vi "dane_do_wykresu.vi"() -> ()   [LabVIEW 2018]
uses:
  <vilib>/Utility/file.llb/Read Delimited Spreadsheet (string).vi
panel:
  out "Mixed Signal Graph":dbl[][](graph)
  in  "Path":path
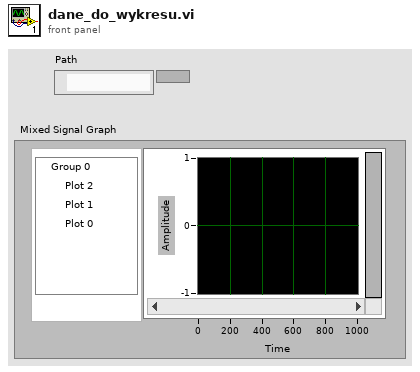
[diagram p1: front panel]
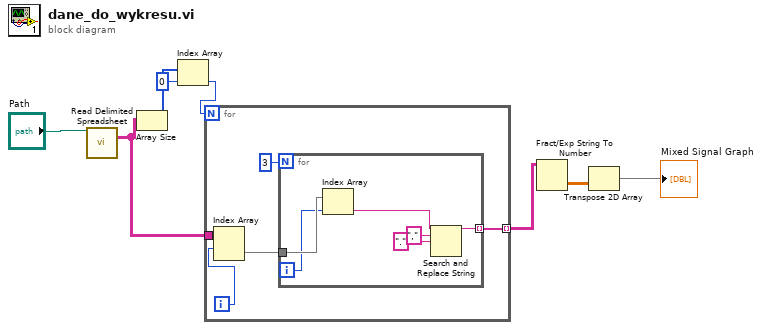
[diagram p0: block diagram]
diagram:
  n1 = call-poly <vilib>:"Read Delimited Spreadsheet.vi"("file path (dialog if empty)"="Path") -> ("all rows"=w2:string[][])  [unwired: 9 in, 5 out]
  n2 = Array Size(array=w2) -> (size(s)=w6:i32[])
  n3 = Index Array(array=w6, index=0) -> (element=w5:i32)
  n4 = for {
    N: w5 -> [_]
    tunnel: [w13] -> w3 mode=indexing
    tunnel: w2 -> [w11]
    i -> [w10]
    n5 = Index Array(array=w11, index (row)=w10) -> (element=w9:string[])  [unwired: 1 in]
    n6 = for {
      N: 3 -> [_]
      tunnel: [w17] -> w13 mode=indexing
      tunnel: w9 -> [w16]
      i -> [w15]
      n7 = Index Array(array=w16, index=w15) -> (element=w14:string)
      n8 = Search and Replace String(input string=w14, search string=",", replace string="." ("replace string (\"\")")) -> (result string=w17:string)  [unwired: 5 in, 3 out]
    }
  }
  n9 = Fract/Exp String To Number(string=w3) -> (number=w7:dbl[][])  [unwired: 3 in, 1 out]
  n10 = Transpose 2D Array(2D array=w7) -> (transposed array=→"Mixed Signal Graph":dbl[][])
